vi "LEDs.vi"   [LabVIEW 2016]
uses:
  <vilib>/Platform/TimedLoop/XDataNode/timing_clust.ctl
  <vilib>/Platform/TimedLoop/XDataNode/nitl_modes.ctl
  <vilib>/Platform/TimedLoop/XDataNode/wakeup.ctl
  <vilib>/rvi/Emulation/niFpgaSctlEmulationGetInTimedLoop.vi
  <vilib>/rvi/Emulation/niFpgaEmulationReportErrorSimple.vi
  <vilib>/rvi/Emulation/niFpgaGetClockAttributes.vi
  <vilib>/rvi/Emulation/niFpgaCriticalErrorInLSC.vi
  <vilib>/rvi/eio/common/nirviEmuTemplateMethod_errors.vi
  <vilib>/Platform/TimedLoop/XDataNode/XDataNode.xnode
  <vilib>/eio/EIONode/EIONode.xnode
  <vilib>/Platform/TimedLoop/XDataNode/XDNodeRunTimeDep.lvlib
types:
  T1 = typedef "XDNodeRunTimeDep.lvlib/timing_clust.ctl" = cluster{"Expected End [f-1]":u64, "Actual End [f-1]":u64, "Finished Late? [f-1]":bool, "Expected End [i-1]":u64, "Actual End [i-1]":u64, "Finished Late? [i-1]":bool, "Expected Start [i]":u64, "Actual Start [i]":u64, "Expected Start [f]":u64, "Actual Start [f]":u64, "Source Name":string, "Structure Name":string, "Period":i64, "Deadline":i64, "Offset":i64, "Start":i64, "Priority":i32, "Timeout":i32, "Mode":T2, "Wakeup Reason":T3, "Error":errorcluster, "Source Type":string, "Secondary Source Type":string, "Global End Time":u64, "Global Start Time":u64, "Frame Duration":u64, "Iteration Duration":u64, "Assigned CPU":i32, "I/O Scan Engine Mode":u32}
  T2 = typedef "XDNodeRunTimeDep.lvlib/nitl_modes.ctl" = enum32{"No Change", "Process missed periods, maintain original phase", "Discard missed periods, maintain original phase", "Process missed periods, ignore original phase", "Discard missed periods, ignore original phase"}
  T3 = typedef "XDNodeRunTimeDep.lvlib/wakeup.ctl" = enum32{"Normal", "Aborted", "Asynchronous wakeup", "Timing source error", "Timed loop error", "Timeout"}
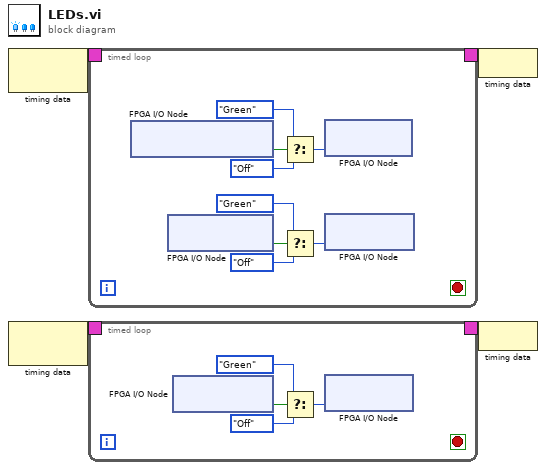
[diagram p0: block diagram]
diagram:
  n1 = node-c288() -> (w4:T1)  [unwired: 1 in]
  n2 = node-c288() -> (w2:T1)  [unwired: 1 in]
  n3 = timed-loop {
    timing: w4 -> [_]
    timing-out: [_] -> w3
    stop <- _ stop-if-true
    n4 = xnode ("FPGA I/O Node")() -> ("Clock Chip Locked"=w5:bool)  [unwired: 1 in, 1 out]
    n5 = xnode ("FPGA I/O Node")() -> ("GPS Locked"=w9:bool)  [unwired: 1 in, 1 out]
    n6 = Select(t=enum8{"Off", "Green"}."Green" ("LED/REF"), s=w5, f=enum8{"Off", "Green"}."Off" ("LED/REF")) -> (s? t:f=w8:enum8{"Off", "Green"})
    n7 = Select(t=enum8{"Off", "Green"}."Green" ("LED/GPS"), s=w9, f=enum8{"Off", "Green"}."Off" ("LED/GPS")) -> (s? t:f=w12:enum8{"Off", "Green"})
    n8 = xnode ("FPGA I/O Node")("LED/REF"=w8) -> ()  [unwired: 1 in, 1 out]
    n9 = xnode ("FPGA I/O Node")("LED/GPS"=w12) -> ()  [unwired: 1 in, 1 out]
  }
  n10 = timed-loop {
    timing: w2 -> [_]
    timing-out: [_] -> w1
    stop <- _ stop-if-true
    n11 = xnode ("FPGA I/O Node")() -> ("PPS Trig In"=w16:bool)  [unwired: 1 in, 1 out]
    n12 = Select(t=enum8{"Off", "Green"}."Green" ("LED/PPS"), s=w16, f=enum8{"Off", "Green"}."Off" ("LED/PPS")) -> (s? t:f=w15:enum8{"Off", "Green"})
    n13 = xnode ("FPGA I/O Node")("LED/PPS"=w15) -> ()  [unwired: 1 in, 1 out]
  }
  n14 = node-c288(w3) -> ()
  n15 = node-c288(w1) -> ()
